vi "dfd_Dummy_CoefBlock.vi"(2 "coefAddr":u16, 3 "coef name control":cluster{"Coef 0":refnum<k21>}, 4 "new coefficient":T1) -> (7 "coefficients":fxp<+/-,16,1>[](array[numeric]) format="%.16g")   [LabVIEW 2017]
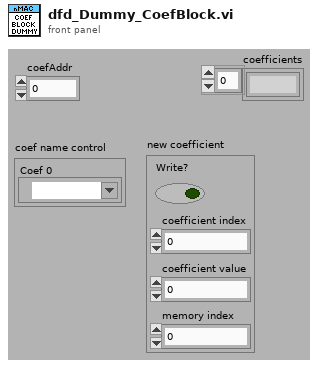
[diagram p1: front panel]
types:
  T1 = cluster{"Write?":bool, "coefficient index":fxp<+/-,16,16>, "coefficient value":fxp<+/-,16,16>, "memory index":fxp<+/-,16,16>}
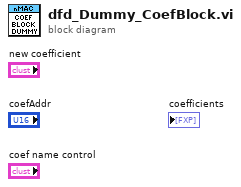
[diagram p0: block diagram]
diagram:
